vi "TEMP MOVE BIAS.vi"(0 "ScanQ in":refnum<queue>, 2 "Translation":cluster{"x":dbl, "y":dbl}, 5 "x":dbl, 7 "Boolean":bool, 9 "y":dbl, 11 "error in (no error)":errorcluster) -> (4 "ScanQ out":refnum<queue>, 6 "X (m)":sgl, 10 "Y (m)":sgl, 15 "error out":errorcluster)   [LabVIEW 2025]
uses:
  Desktop/STM-Auto-Project/QMH CTLS/Scan_Params (QMH).ctl
  Desktop/Magnetic Drift Correction/Bias Cont QMH.ctl
panel:
  in  "Bias in":T1 {"Final Y (m)" format="%.3p"; "Final X (m)" format="%.3p"}
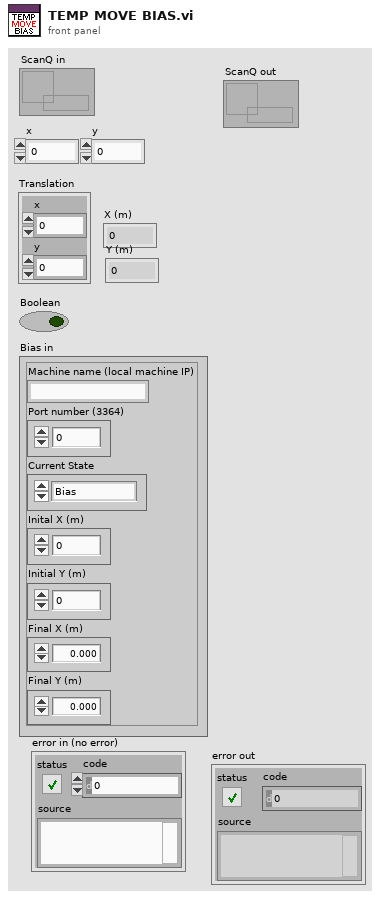
[diagram p1: front panel]
types:
  T1 = typedef "Bias Cont QMH.ctl" = cluster{"Machine name (local machine IP)":string, "Port number (3364)":u32, "Current State":enum16{"Bias", "Stop"}, "Inital X (m)":dbl, "Initial Y (m)":dbl, "Final X (m)":sgl, "Final Y (m)":sgl}
  T2 = enum16{"1. BIAS", "2. INIT_SCAN", "3. SCAN_IDLE", "4. INTER_SCAN", "5. NEW_COORDS_&_FRAME", "6. FINAL_SCAN", "7. POLL BIAS ", "8. Z-CONT.", "9. STOP"}
  T3 = typedef "Scan_Params (QMH).ctl" = cluster{"Setpoint (I)":dbl[], "Bias (V)":dbl[], "Number of scans":u8, "Port number (3364)":u32, "Avoid zero threshold (V)":dbl, "Current State":enum16{"1. BIAS", "2. INIT_SCAN", "3. SCAN_IDLE", "4. INTER_SCAN", "5. NEW_COORDS_&_FRAME", "6. FINAL_SCAN", "7. POLL BIAS ", "8. Z-CONT.", "9. STOP"}}
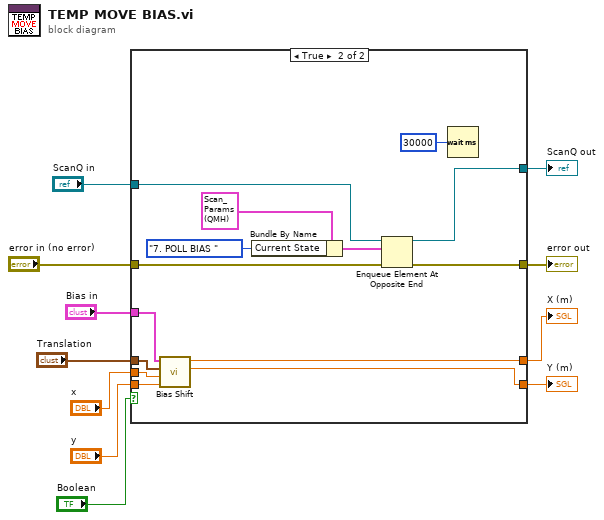
[diagram p0: block diagram]
diagram:
  n1 = case shown="True" "Boolean" {
    tunnel: "Translation" -> [_ w24]
    tunnel: "ScanQ in" -> [w15 w27]
    tunnel: [w15 w28] -> w8
    tunnel: [w14 w17] -> w9
    tunnel: "error in (no error)" -> [w14 w25]
    tunnel: [w13 w23] -> w4
    tunnel: "Bias in" -> [_ w22]
    tunnel: [w12 w20] -> w3
    tunnel: "x" -> [w13 w19]
    tunnel: "y" -> [w12 w18]
    frame False {
    }
    frame True {
      n2 = call "Bias Shift.vi"("y"=w18, "x"=w19, "Translation (m)"=w24, "Bias Controller"=w22) -> ("Y (m)"=w20:sgl, "X (m)"=w23:sgl)  [unwired: 6 in]
      n3 = Bundle By Name(cluster=T3 {"Setpoint (I)"=[], "Bias (V)"=[], "Number of scans"=1, "Port number (3364)"=3364, "Avoid zero threshold (V)"=0.004999999888241291, "Current State"=enum."1. BIAS"} ("element"), "Current State"=T2."7. POLL BIAS ") -> (w21:T3)
      n4 = Enqueue Element At Opposite End(queue=w27, element=w21, error in (no error)=w25) -> (queue out=w28:refnum<queue>, error out=w17:errorcluster)  [unwired: 1 in, 1 out]
      n5 = Wait (ms)(milliseconds to wait=u32 30000) -> ()  [unwired: 1 out]
    }
  }
  "error out" <- w9
  "ScanQ out" <- w8
  "X (m)" <- w4
  "Y (m)" <- w3
